vi "test.vi"() -> ()   [LabVIEW 2015]
panel:
  out "Numeric":dbl
  in  "Array 2":dbl[](array[numeric])
  out "Array":dbl[](array[numeric])
  in  "Threshold":dbl
  in  "Number of elements":dbl
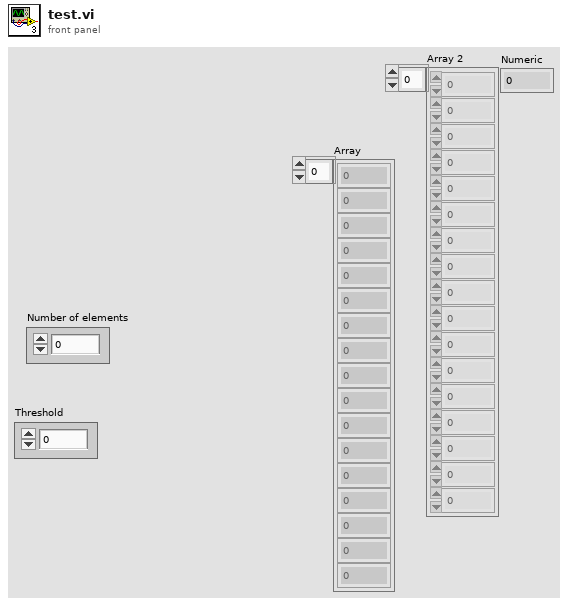
[diagram p1: front panel]
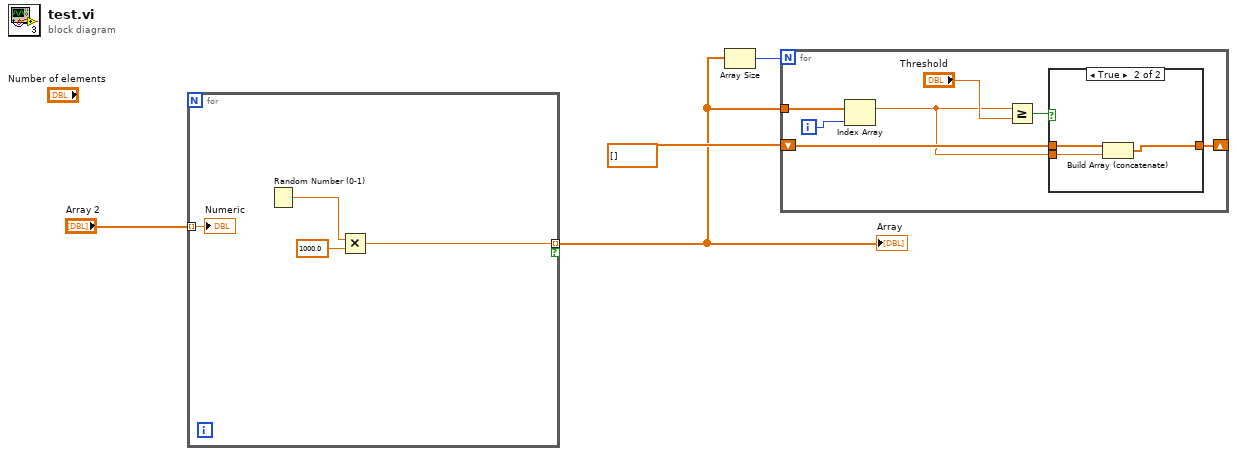
[diagram p0: block diagram]
diagram:
  n1 = for {
    tunnel: [w6] -> w1 mode=indexing if=_
    tunnel: "Array 2" -> [w5] mode=indexing
    n2 = Random Number (0-1)() -> (number: 0 to 1=w8:dbl)
    n3 = Multiply(x=w8, y=1000.0) -> (x*y=w6:dbl)
    "Numeric" <- w5
  }
  "Array" <- w1
  n4 = Array Size(array=w1) -> (size(s)=w2:i32)
  n5 = for {
    N: w2 -> [_]
    tunnel: w1 -> [w12]
    shift-right: [w11] -> _
    shift-left: dbl[] [] -> [w13]
    i -> [w9]
    n6 = Index Array(array=w12, index=w9) -> (element=w10:dbl)
    n7 = Greater Or Equal?(x=w10, y="Threshold") -> (x >= y?=w14:bool)
    n8 = case shown="True" w14 {
      tunnel: w13 -> [w16 w19]
      tunnel: w10 -> [_ w18]
      tunnel: [w16 w17] -> w11
      frame False {
      }
      frame True {
        n9 = Build Array (concatenate)(w19, w18) -> (w17:dbl[])
      }
    }
  }
